vi "Create.vi"(6 "chunk size":u64=4000, 8 "error in (no error)":errorcluster, 9 "operation (0: open or create)":T1, 10 "stream mode (0: File)":T3, 11 "file":path) -> (0 "error out":errorcluster, 3 "Excel refnum out":T2)   [LabVIEW 2017, in "NI_ExcelFile.lvlib"]
doc: "Creates a .xlsx file for writing. You can also use this VI to open or replace an existing .xlsx file that you created by using the Write To Measurement File Express VI or this VI. Use the Destroy VI to close the reference to the file.\n \nfile: Specifies the absolute path to the file you want to create. The file extension of the filename you specify in file must be .xlsx .Otherwise, you can not open the file in Excel.\nstream mode: Specifies the mode this VI uses to stream the data to the .xlsx file.\n0 File- Costs less memory but is slower than Memory mode.\n1 Memory- Costs more memory but is faster than File mode.\n\noperation: specifies the operation to perform. \n0 open or create (default)-Creates a new .xlsx file or opens an existing .xlsx file to configure.\n1 create-Creates a new .xlsx file.\n2 create or replace-Creates a new .xlsx file or replaces an existing .xlsx file.\n3 open-Opens a .xlsx file to write to. \n\nchunk size : Specifies the size of each chunk of data that this VI writes data to the .xlsx file.\n\nerror in: describes error conditions that occur before this node runs. This input provides standard error in functionality.\n\nExcel refnum out: Returns a Microsoft Excel file reference to the .xlsx file on which you performed the operation.\n\nerror out: contains error information. This output provides standard error out functionality."
uses:
  <vilib>/express/express shared/NI_ExcelFile/NI_ExcelFile.lvlib
  <vilib>/express/express shared/NI_ExcelFile/Ctrls/StreamMode.ctl
  <vilib>/express/express shared/NI_ExcelFile/Ctrls/ExcelRefnum.ctl
  <vilib>/express/express shared/NI_ExcelFile/Ctrls/MainData.ctl
  <vilib>/express/express shared/NI_ExcelFile/Ctrls/TimeColumnMode.ctl
  <vilib>/express/express shared/NI_ExcelFile/Ctrls/FileAttribute.ctl
  <vilib>/express/express shared/NI_ExcelFile/Ctrls/Columns.ctl
  <vilib>/express/express shared/NI_ExcelFile/Ctrls/ColumnInfo.ctl
  <vilib>/express/express shared/NI_ExcelFile/Ctrls/DataType.ctl
  <vilib>/express/express shared/NI_ExcelFile/Ctrls/wd_recordInfo.ctl
  <vilib>/express/express shared/NI_ExcelFile/Ctrls/disk_TemplateFile.ctl
  <vilib>/express/express shared/NI_ExcelFile/Ctrls/meta_file.ctl
  <vilib>/express/express shared/NI_ExcelFile/Ctrls/meta_Block.ctl
  <vilib>/express/express shared/NI_ExcelFile/Ctrls/meta_BlockType.ctl
  <vilib>/express/express shared/NI_ExcelFile/Ctrls/FileOperation.ctl
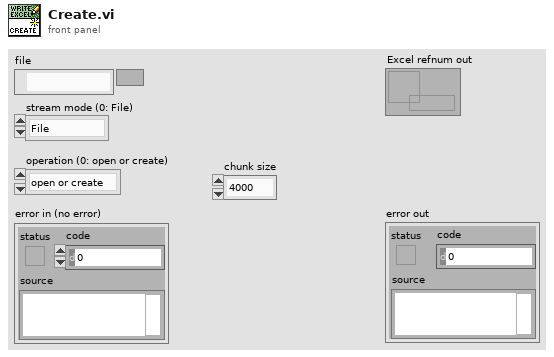
[diagram p1: front panel]
types:
  T1 = typedef "NI_ExcelFile.lvlib/FileOperation.ctl" = enum16{"open or create", "open", "create or replace", "create"}
  T2 = typedef "NI_ExcelFile.lvlib/ExcelRefnum.ctl" = refnum<data-value>
  T3 = typedef "NI_ExcelFile.lvlib/StreamMode.ctl" = enum16{"File", "Memory"}
  T4 = typedef "NI_ExcelFile.lvlib/MainData.ctl" = cluster{"TargetFile":path, "StreamMode":T3, "Append?":bool, "ChunkSize":u64, "TimeColumnMode":T5, "TimestampFormat":string, "AbsoluteTime?":bool, "FileAttribute ":T6, "Column":T7, "FileRef":refnum<k1>, "MemoryRef":refnum<data-value>[], "RecordInfo":T10[], " ChannelPreviousInfo":u32[], "ChannelFirstRecord":u32[], "PredefinedFormattedValueLength":i64, "DiskTemplate":T11}
  T5 = typedef "NI_ExcelFile.lvlib/TimeColumnMode.ctl" = enum16{"Empty", "OnePerCh", "One"}
  T6 = typedef "NI_ExcelFile.lvlib/FileAttribute.ctl" = cluster{"Creator":string, "Title":string, "SheetName":string}
  T7 = typedef "NI_ExcelFile.lvlib/Columns.ctl" = T8[]
  T8 = typedef "NI_ExcelFile.lvlib/ColumnInfo.ctl" = cluster{"Header":string, "Format":string, "DataType":T9, "Length":u64}
  T9 = typedef "NI_ExcelFile.lvlib/DataType.ctl" = enum16{"DDT", "WFM", "Array of STR", "Array of DBL", "Array of I8", "Array of I16", "Array of I32", "Array of I64", "Array of SGL", "Array of U8", "Array of U16", "Array of U32", "Array of U64", "Array of Time"}
  T10 = typedef "NI_ExcelFile.lvlib/wd_recordInfo.ctl" = cluster{"ChannelIndex":u32, "StartIndex":u64, "Length":u64, "Previous":i32, "Next":i32}
  T11 = typedef "NI_ExcelFile.lvlib/disk_TemplateFile.ctl" = cluster{"XMLRef":refnum<file>[], "ZipPath":path, "MetaFile":T12, "TempFolder":path}
  T12 = typedef "NI_ExcelFile.lvlib/meta_file.ctl" = cluster{"Ref":refnum<file>, "NextRow":i32, "NextPosition":i64, "Block":T13[]}
  T13 = typedef "NI_ExcelFile.lvlib/meta_Block.ctl" = cluster{"Version":u16, "Type":T14, "Length":i32, "Data":string}
  T14 = typedef "NI_ExcelFile.lvlib/meta_BlockType.ctl" = enum16{"NITag", "File", "Column"}
  T15 = enum16{"open", "replace", "create", "open or create", "replace or create", "replace or create with confirmation"}
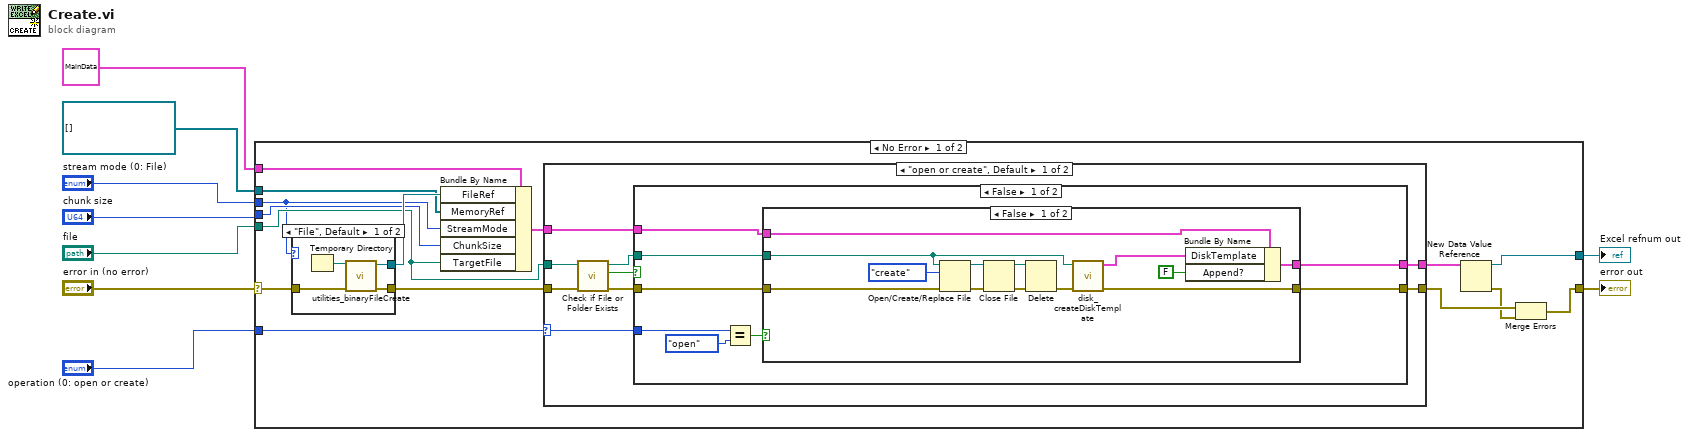
[diagram p0: block diagram]
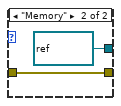
[diagram p2: hidden frame]
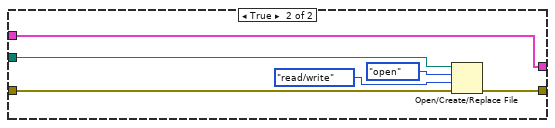
[diagram p3: hidden frame]
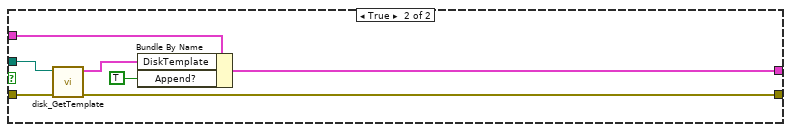
[diagram p4: hidden frame]
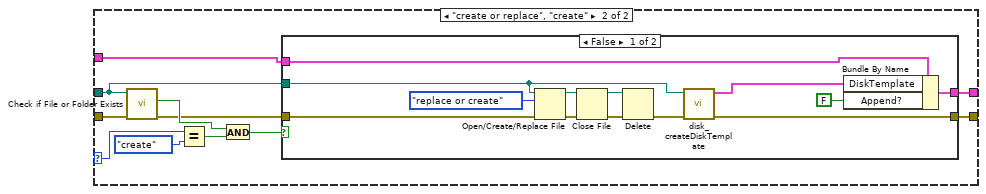
[diagram p5: hidden frame]
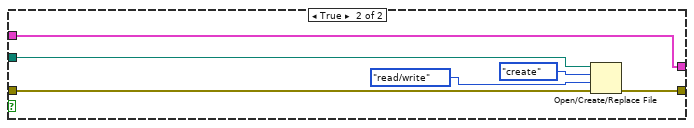
[diagram p6: hidden frame]
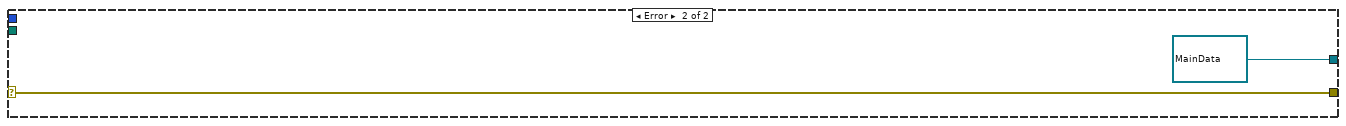
[diagram p7: hidden frame]
diagram:
  n1 = case shown="No Error" "error in (no error)" {
    selector: "error in (no error)" -> [w15 w105]
    tunnel: "stream mode (0: File)" -> [w13 _]
    tunnel: [w10 w105] -> w8
    tunnel: "chunk size" -> [w23 _]
    tunnel: [w21 refnum<data-value> refnum ("data value reference")] -> w6
    tunnel: refnum<data-value>[] [] ("MemoryRef") -> [w20 _]
    tunnel: "operation (0: open or create)" -> [w19 _]
    tunnel: "file" -> [w17 _]
    tunnel: T4 {"TargetFile"=path "", "StreamMode"=enum."File", "Append?"=FALSE, "ChunkSize"=0, "TimeColumnMode"=enum."Empty", "TimestampFormat"="", "AbsoluteTime?"=FALSE, "FileAttribute "={"Creator"="", "Title"="", "SheetName"=""}, "Column"=[], "FileRef"=refnum, "MemoryRef"=[], "RecordInfo"=[], " ChannelPreviousInfo"=[], "ChannelFirstRecord"=[], "PredefinedFormattedValueLength"=20, "DiskTemplate"={"XMLRef"=[refnum, refnum, refnum, refnum, refnum, refnum], "ZipPath"=path "", "MetaFile"={"Ref"=refnum, "NextRow"=0, "NextPosition"=0, "Block"=[]}, "TempFolder"=path ""}} ("MainData") -> [w16 _]
    frame No Error {
      n2 = case shown="\"File\", Default" w13 {
        tunnel: [w27 refnum<k1> refnum ("refnum out")] -> w24
        tunnel: w15 -> [w26 w29]
        tunnel: [w25 w29] -> w14
        frame "File", Default {
          n3 = Temporary Directory() -> (w28:path)
          n4 = call <vilib>:"utilities_binaryFileCreate.vi"("error in (no error)"=w26, "path"=w28) -> ("error out"=w25:errorcluster, "refnum out"=w27:refnum<k1>)  [unwired: 8 in]
        }
        frame "Memory" {
        }
      }
      n5 = Bundle By Name(cluster=w16, "FileRef"=w24, "MemoryRef"=w20, "StreamMode"=w13, "ChunkSize"=w23, "TargetFile"=w17) -> (w18:T4)
      n6 = case shown="\"open or create\", Default" w19 {
        selector: w19 -> [w31 w80]
        tunnel: w17 -> [w37 w81]
        tunnel: w14 -> [w39 w75]
        tunnel: w18 -> [w35 w84]
        tunnel: [w34 w83] -> w22
        tunnel: [w33 w82] -> w12
        frame "open or create", Default {
          n7 = call <vilib>:"Check if File or Folder Exists.vi"("error in (no error)"=w39, "path"=w37) -> ("error out"=w36:errorcluster, "file or folder exists?"=w38:bool, "dup path"=w32:path)  [unwired: 7 in]
          n8 = case shown="False" w38 {
            tunnel: w36 -> [w47 w71]
            tunnel: w35 -> [w46 w73]
            tunnel: [w45 w72] -> w34
            tunnel: [w43 w69] -> w33
            tunnel: w32 -> [w44 w70]
            tunnel: w31 -> [w42 _]
            frame False {
              n9 = Equal?(x=w42, y=FileOperation."open" ("operation (0:open or replace)")) -> (x = y?=w40:bool)
              n10 = case shown="False" w40 {
                tunnel: w47 -> [w50 w63]
                tunnel: w46 -> [w60 w66]
                tunnel: [w55 w66] -> w45
                tunnel: w44 -> [w56 w61]
                tunnel: [w48 w62] -> w43
                frame False {
                  n11 = Open/Create/Replace File(file path (use dialog)=w56, error in=w50, operation (0:open)=T15."create") -> (refnum out=w53:refnum<file>, error out=w54:errorcluster)  [unwired: 3 in, 1 out]
                  n12 = Close File(refnum=w53, error in=w54) -> (path=w51:path, error out=w52:errorcluster)
                  n13 = Delete(path (use dialog)=w51, error in=w52) -> (error out=w49:errorcluster)  [unwired: 3 in, 2 out]
                  n14 = call <vilib>:"disk_createDiskTemplate.vi"("error in (no error)"=w49, "File path"=w56) -> ("error out"=w48:errorcluster, "output cluster"=w58:T11)  [unwired: 8 in]
                  n15 = Bundle By Name(cluster=w60, "DiskTemplate"=w58, "Append?"=FALSE ("Append")) -> (w55:T4)
                }
                frame True {
                  n16 = Open/Create/Replace File(file path (use dialog)=w61, error in=w63, operation (0:open)=T15."open", access (0:read/write)=enum16{"read/write", "read-only", "write-only"}."read/write") -> (error out=w62:errorcluster)  [unwired: 2 in, 2 out]
                }
              }
            }
            frame True {
              n17 = call <vilib>:"disk_GetTemplate.vi"("error in (no error)"=w71, "file path"=w70) -> ("error out"=w69:errorcluster, "DiskTemplate"=w67:T11)  [unwired: 8 in]
              n18 = Bundle By Name(cluster=w73, "DiskTemplate"=w67, "Append?"=TRUE ("Append")) -> (w72:T4)
            }
          }
        }
        frame "create or replace", "create" {
          n19 = call <vilib>:"Check if File or Folder Exists.vi"("error in (no error)"=w75, "path"=w81) -> ("error out"=w74:errorcluster, "file or folder exists?"=w78:bool)  [unwired: 7 in, 1 out]
          n20 = Equal?(x=w80, y=FileOperation."create" ("operation (0:open or replace)")) -> (x = y?=w77:bool)
          n21 = And(x=w78, y=w77) -> (x .and. y?=w76:bool)
          n22 = case shown="False" w76 {
            tunnel: w74 -> [w87 w100]
            tunnel: w84 -> [w97 w103]
            tunnel: [w92 w103] -> w83
            tunnel: [w85 w99] -> w82
            tunnel: w81 -> [w93 w102]
            frame False {
              n23 = Open/Create/Replace File(file path (use dialog)=w93, error in=w87, operation (0:open)=T15."replace or create") -> (refnum out=w88:refnum<file>, error out=w91:errorcluster)  [unwired: 3 in, 1 out]
              n24 = Close File(refnum=w88, error in=w91) -> (path=w89:path, error out=w90:errorcluster)
              n25 = Delete(path (use dialog)=w89, error in=w90) -> (error out=w86:errorcluster)  [unwired: 3 in, 2 out]
              n26 = call <vilib>:"disk_createDiskTemplate.vi"("error in (no error)"=w86, "File path"=w93) -> ("error out"=w85:errorcluster, "output cluster"=w96:T11)  [unwired: 8 in]
              n27 = Bundle By Name(cluster=w97, "DiskTemplate"=w96, "Append?"=FALSE ("Append")) -> (w92:T4)
            }
            frame True {
              n28 = Open/Create/Replace File(file path (use dialog)=w102, error in=w100, operation (0:open)=T15."create", access (0:read/write)=enum16{"read/write", "read-only", "write-only"}."read/write") -> (error out=w99:errorcluster)  [unwired: 2 in, 2 out]
            }
          }
        }
      }
      n29 = New Data Value Reference(data value=w22) -> (data value reference=w21:refnum<data-value>, error out=w11:errorcluster)  [unwired: 1 in]
      n30 = Merge Errors(w12, w11) -> (w10:errorcluster)
    }
    frame Error {
    }
  }
  "error out" <- w8
  "Excel refnum out" <- w6
